vi "AMI.vi"(1 "输入原消息代码":u32[](array[numeric])) -> (0 "变换后的AMI码":i8[](array[numeric]))   [LabVIEW 2013]
uses:
  <vilib>/express/express analysis/Spectral/Block/exnSpectralBlock spectral measurements PSD poly.vi
  <vilib>/express/express analysis/Spectral/Block/exnSpectralBlock spectral measurements PSD WFM.vi
  <vilib>/express/express analysis/Spectral/XNode/ExpressSpectralMeasurementsBlockNode.xnode
panel:
  out "AMI码功率谱密度":cluster{"f0":dbl, "df":dbl, "magnitude":dbl[]}(graph)
  in  "计交替次数":u8
  out "AMI码波形":i32[](graph)
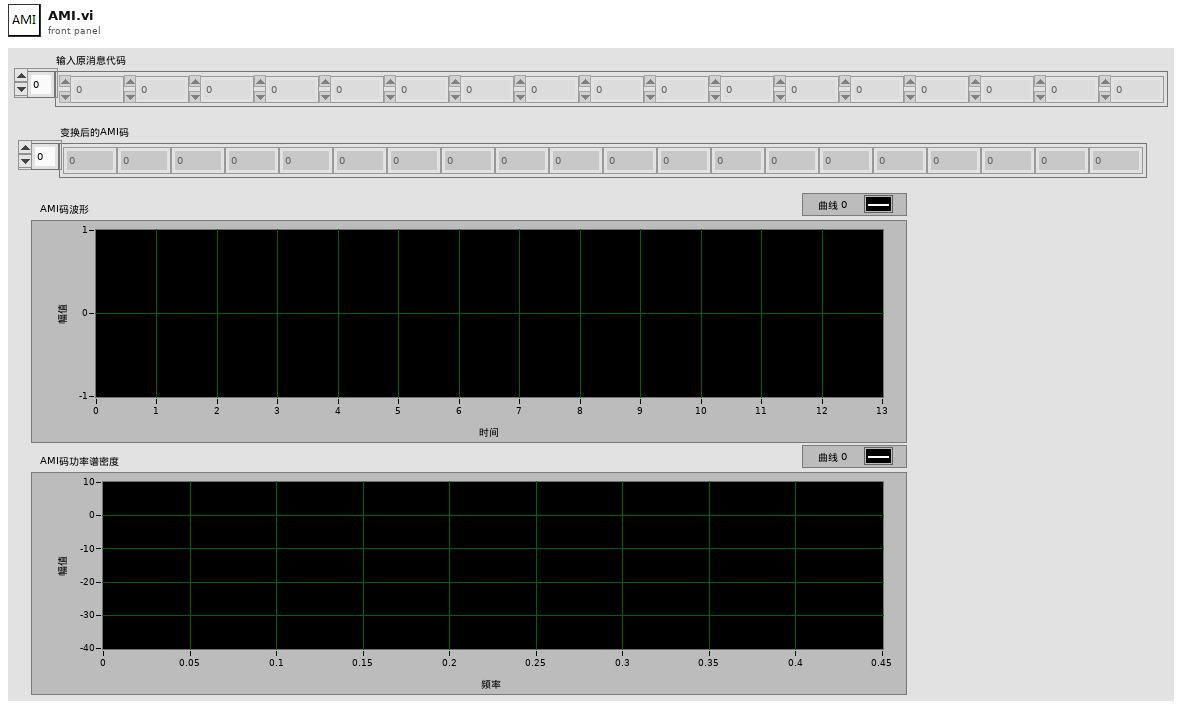
[diagram p1: front panel]
types:
  T1 = cluster{"averaging mode":u16, "weighting mode":u16, "number of averages":u32}
  T2 = cluster{"dB On (F)":bool, "unwrap phase (F)":bool, "convert to degree (F)":bool}
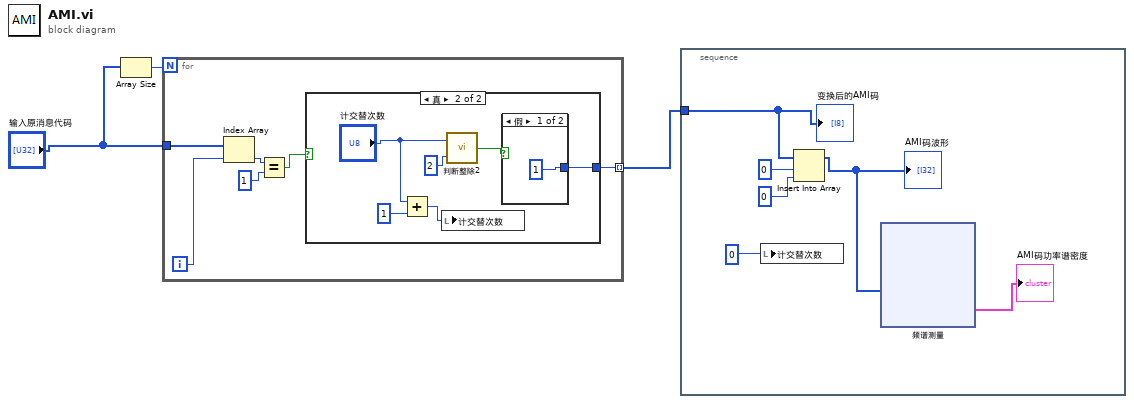
[diagram p0: block diagram]
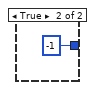
[diagram p3: hidden frame]
diagram:
  n1 = Array Size(array="输入原消息代码") -> (size(s)=w3:i32)
  n2 = for {
    N: w3 -> [_]
    tunnel: "输入原消息代码" -> [w9]
    tunnel: [w4] -> w1 mode=indexing
    i -> [w8]
    n3 = Index Array(array=w9, index=w8) -> (element=w7:u32)
    n4 = Equal?(x=w7, y=1) -> (x = y?=w5:bool)
    n5 = case shown="真" w5 {
      tunnel: [_ w13] -> w4
      frame False {
      }
      frame True {
        n6 = Add(x="计交替次数", y=1) -> (x+y=w10:i32)
        n7 = local write "计交替次数"(w10) -> ()
        n8 = call "判断整除2.vi"("被除数"=2, "除数"="计交替次数") -> ("布尔 2"=w14:bool)
        n9 = case shown="假" w14 {
          tunnel: [1 -1] -> w13
          frame False {
          }
          frame True {
          }
        }
      }
    }
  }
  n10 = stacked-sequence {
    tunnel: w1 -> [w23]
    frame #0 {
      n11 = local write "计交替次数"(0) -> ()
      n12 = Insert Into Array(array=w23, index=0, new element=0) -> (w19:i32[])
      "AMI码波形" <- w19
      n13 = xnode "频谱测量"("信号"=w19) -> ("PSD"=→"AMI码功率谱密度":cluster{"f0":dbl, "df":dbl, "magnitude":dbl[]})  [unwired: 1 in, 1 out]
      "变换后的AMI码" <- w23
    }
  }
